vi "Read Rules.vi"(8 "error in (no error)":errorcluster, 11 "LogFilter In":refnum<class "LogFilter.lvclass">) -> (0 "error out":errorcluster, 2 "Rules":T1={"Global"={"CSM"=[], "LogType"=[], "State"=[], "StateType"=[], "Broadcast"=[], "UserLog"=[]}, "CSM"={"LogType"=[], "State"=[], "StateType"=[], "Broadcast"=[], "UserLog"=[]}, "PeriodicMessageFilter"={"Enable"=FALSE, "Threshold(#/s)"=1.0, "CheckPeriod(s)"=1.0}}, 3 "LogFilter Out":refnum<class "LogFilter.lvclass">)   [LabVIEW 2017, in "Communicable State Machine.lvlib" / "LogFilter.lvclass"]
uses:
  LogFilter.lvclass
  Typedef/_CSM_GlobalLog Filter Rules - v1.2.ctl
  Typedef/_CSM_GlobalLog_MSG_TYPE.ctl
  Typedef/_CSM_GlobalLog_STATE_TYPE.ctl
  LogFilter.lvclass/LogFilter.ctl
  Communicable State Machine.lvlib
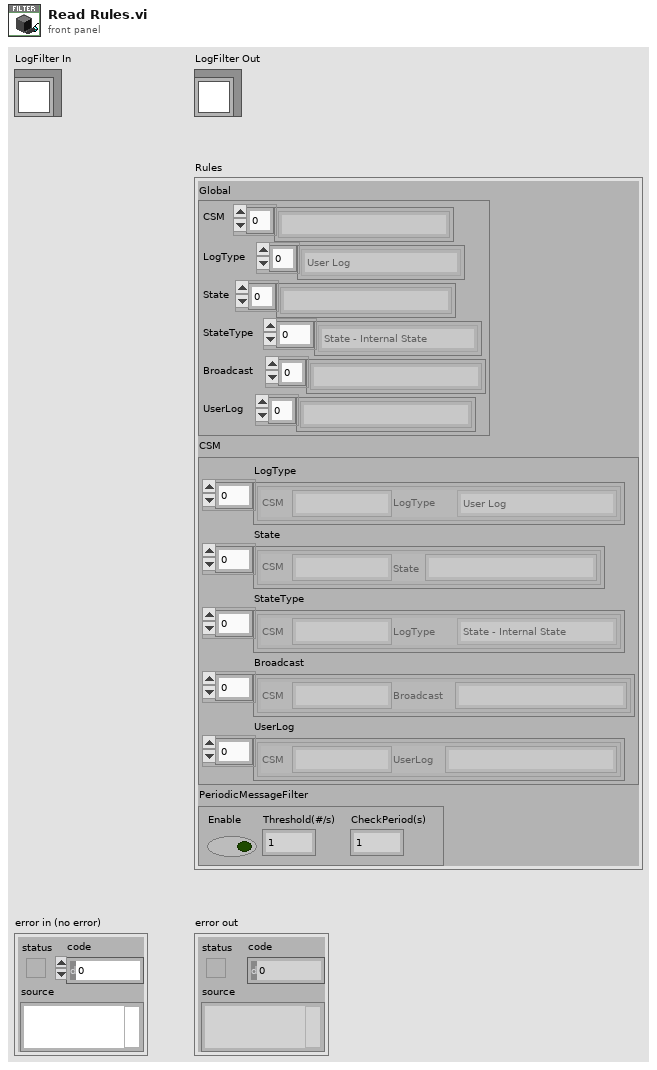
[diagram p1: front panel]
types:
  T1 = typedef "Communicable State Machine.lvlib/_CSM_GlobalLog Filter Rules - v1.2.ctl" = cluster{"Global":cluster{"CSM":string[], "LogType":T2[], "State":string[], "StateType":T3[], "Broadcast":string[], "UserLog":string[]}, "CSM":cluster{"LogType":cluster{"CSM":string, "LogType":T2}[], "State":cluster{"CSM":string, "State":string}[], "StateType":cluster{"CSM":string, "LogType":T3}[], "Broadcast":cluster{"CSM":string, "Broadcast":string}[], "UserLog":cluster{"CSM":string, "UserLog":string}[]}, "PeriodicMessageFilter":cluster{"Enable":bool, "Threshold(#/s)":dbl, "CheckPeriod(s)":dbl}}
  T2 = typedef "Communicable State Machine.lvlib/_CSM_GlobalLog_MSG_TYPE.ctl" = enum16{"User Log", "State Change", "Status", "Interrupt", "Register", "Unregister", "Error Log", "Module Created", "Module Destroyed", "Async Message", "No-Rep Async Message", "Sync Message", "AsyncMsg Complete", "SyncMsg Complete"}
  T3 = typedef "Communicable State Machine.lvlib/_CSM_GlobalLog_STATE_TYPE.ctl" = enum16{"State - Internal State", "State - External Message", "State - Response", "State - Complete"}
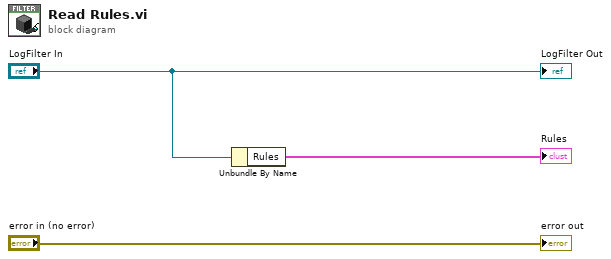
[diagram p0: block diagram]
diagram:
  n1 = Unbundle By Name("LogFilter In") -> ("Rules"=→"Rules":T1)
  "error out" <- "error in (no error)"
  "LogFilter Out" <- "LogFilter In"
